vi "ImportSession.vi"(8 "error in (no error)":errorcluster, 9 "Clust Refnum":refnum<vi>, 11 "Database in":refnum<class "Database.lvclass">) -> (0 "error out":errorcluster, 1 "Clust Refnum 2":refnum<vi>, 3 "Database out":refnum<class "Database.lvclass">)   [LabVIEW 2014, in "Database.lvclass"]
uses:
  Database.lvclass
  Database.lvclass/Database.ctl
  <vilib>/addons/database/NI_Database_API.lvlib
panel:
  in  "Value":variant
  in  "session":T1
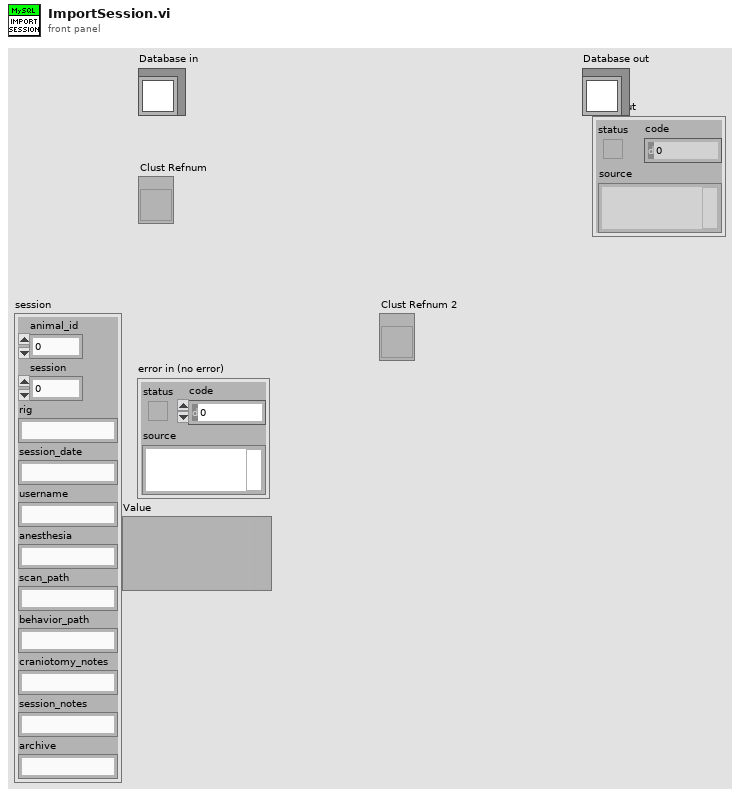
[diagram p1: front panel]
types:
  T1 = cluster{"animal_id":dbl, "session":dbl, "rig":string, "session_date":string, "username":string, "anesthesia":string, "scan_path":string, "behavior_path":string, "craniotomy_notes":string, "session_notes":string, "archive":string}
  T2 = typedef "NI_Database_API.lvlib/Conn ObjectReference.ctl" = refnum<k1>
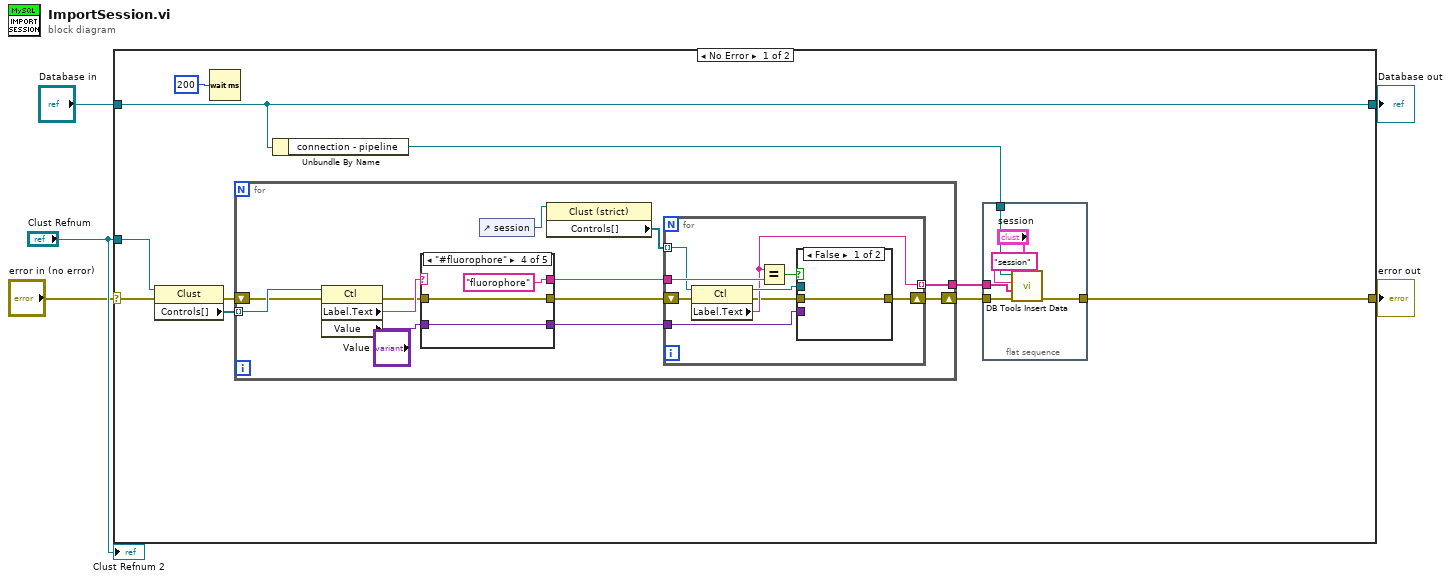
[diagram p0: block diagram]
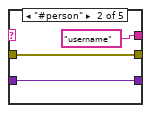
[diagram p3: hidden frame]
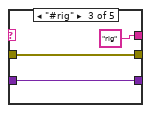
[diagram p4: hidden frame]
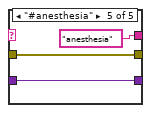
[diagram p5: hidden frame]
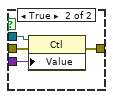
[diagram p6: hidden frame]
diagram:
  n1 = case shown="No Error" "error in (no error)" {
    selector: "error in (no error)" -> [w12 w63]
    tunnel: [w11 w64] -> w2
    tunnel: "Database in" -> [w11 w64]
    tunnel: "Clust Refnum" -> [w14 _]
    tunnel: [w6 w63] -> w1
    frame No Error {
      n2 = property class="Clust"(reference=w14, error in=w12) -> (error out=w13:errorcluster, "Controls[]"=w15:refnum<vi>[])  [unwired: 1 out]
      n3 = Wait (ms)(milliseconds to wait=u32 200) -> ()  [unwired: 1 out]
      n4 = for {
        tunnel: w15 -> [w33] mode=indexing
        shift-right: [w25] -> w8
        shift-left: w13 -> [w32]
        tunnel: [w29] -> w10
        n5 = property class="Ctl"(reference=w33, error in=w32) -> (error out=w27:errorcluster, "Label.Text"=w28:string, "Value"=w24:variant)  [unwired: 1 out]
        n6 = case shown="\"#fluorophore\"" w28 {
          selector: w28 -> [w36 _ _ _ _]
          tunnel: [w36 "username" ("session") "rig" ("session") "fluorophore" ("session") "anesthesia"] -> w22
          tunnel: w27 -> [w35 w37 w40 w44 w47]
          tunnel: [w35 w37 w40 w44 w47] -> w26
          tunnel: w24 -> [w34 w38 w41 w43 w46]
          tunnel: [w34 w38 w41 w43 w46] -> w23
          frame "False", Default {
          }
          frame "#person" {
          }
          frame "#rig" {
          }
          frame "#fluorophore" {
          }
          frame "#anesthesia" {
          }
        }
        n7 = control-ref of="session"() -> (w31:refnum<vi>)
        n8 = property class="Clust (strict)"(reference=w31) -> ("Controls[]"=w30:refnum<vi>[])  [unwired: 1 in, 2 out]
        n9 = for {
          tunnel: w22 -> [w57]
          tunnel: w23 -> [w54]
          tunnel: w30 -> [w56] mode=indexing
          tunnel: [w52] -> w29 mode=indexing
          shift-right: [w49] -> w25
          shift-left: w26 -> [w51]
          n10 = property class="Ctl"(reference=w56, error in=w51) -> (reference out=w55:refnum<vi>, error out=w50:errorcluster, "Label.Text"=w52:string)
          n11 = Equal?(x=w52, y=w57) -> (x = y?=w53:bool)
          n12 = case shown="False" w53 {
            tunnel: w55 -> [_ w62]
            tunnel: w54 -> [_ w61]
            tunnel: w50 -> [w58 w60]
            tunnel: [w58 w59] -> w49
            frame False {
            }
            frame True {
              n13 = property class="Ctl"(reference=w62, error in=w60, "Value"=w61) -> (error out=w59:errorcluster)  [unwired: 1 out]
            }
          }
        }
      }
      n14 = Unbundle By Name(w11) -> ("connection - pipeline"=w9:T2)
      n15 = flat-sequence {
        tunnel: w10 -> [w21]
        tunnel: w9 -> [w20]
        tunnel: w8 -> [w19]
        tunnel: [w17] -> w6
        frame #0 {
          n16 = call <vilib>:"DB Tools Insert Data.vi"("data"="session", "error in (no error)"=w19, "columns"=w21, "table"="session" ("session"), "connection reference"=w20) -> ("error out"=w17:errorcluster)  [unwired: 5 in, 1 out]
        }
      }
    }
    frame Error {
    }
  }
  "error out" <- w1
  "Database out" <- w2
  "Clust Refnum 2" <- "Clust Refnum"
